vi "WaveFormnew.vi"(11 "2D Double Array 3":i32[][](array[numeric])) -> (1 "2D Double Array":i32[](array[numeric]), 2 "Waveform Chart 3":waveform(i32)[](graph) caption="Waveform Chart 2", 3 "2D Double Array 2":i32[][](array[numeric]), 4 "Waveform Chart":waveform(i32)(graph), 5 "XY Graph":cluster{i32[], u64[]}(graph))   [LabVIEW 2023]
uses:
  <vilib>/numeric/Random Number (Range) U64.vi
  <vilib>/numeric/sub_Random U32.vi
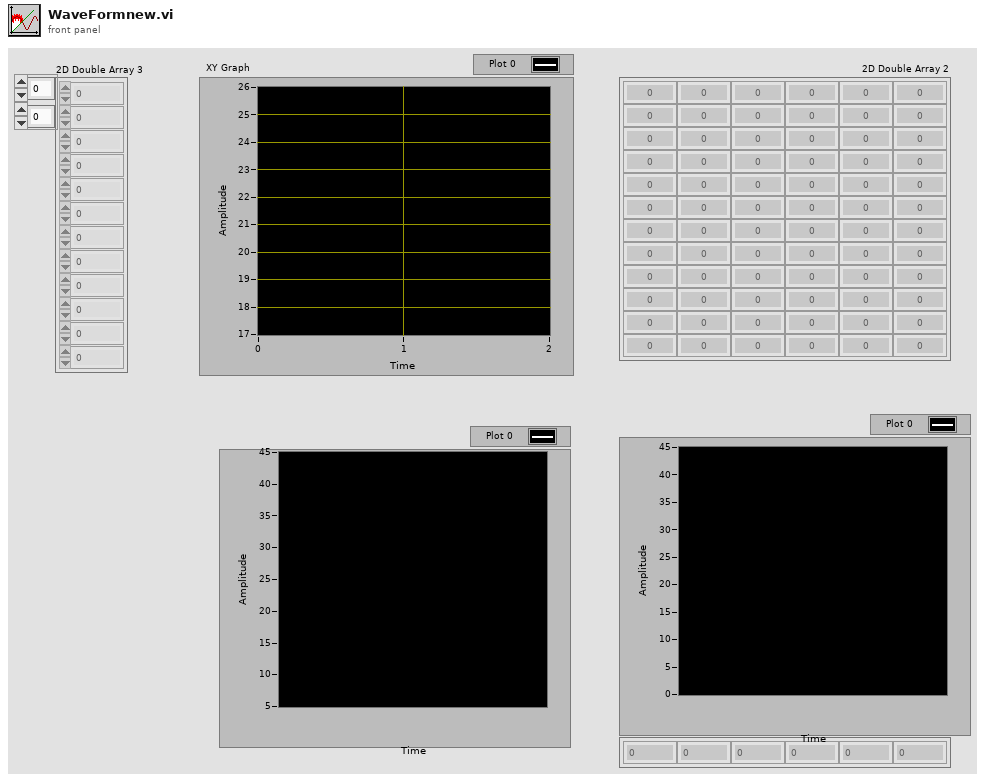
[diagram p1: front panel]
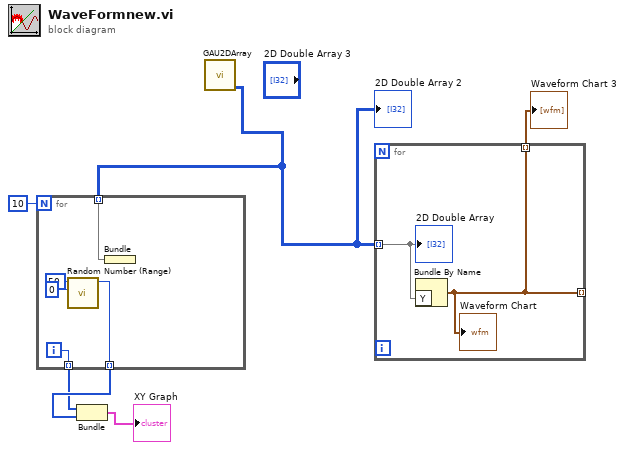
[diagram p0: block diagram]
diagram:
  n1 = call "GAU2DArray.vi"() -> ("2D Double Array"=w1:i32[][])  [unwired: 10 in, 1 out]
  "2D Double Array 2" <- w1
  n2 = for {
    N: 10 -> [_]
    tunnel: w1 -> [w11] mode=indexing
    tunnel: [w10] -> w3 mode=indexing
    tunnel: [w7] -> w4 mode=indexing
    i -> [w10]
    n3 = call-poly <vilib>:"Random Number (Range).vi"("lower bound (0)"=u64 0, "upper bound (100)"=u64 50) -> ("number"=w7:u64)  [unwired: 9 in]
    n4 = Bundle("2D Double Array"=w11) -> ()  [unwired: 1 in, 1 out]
  }
  n5 = Bundle(w3, w4) -> (→"XY Graph":cluster{i32[], u64[]})  [unwired: 1 in]
  n6 = for {
    tunnel: w1 -> [w13] mode=indexing
    tunnel: [w12] -> _ mode=indexing
    tunnel: [w12] -> w2 mode=indexing
    n7 = Bundle By Name("Y"=w13) -> (w12:waveform(i32))  [unwired: 1 in]
    "Waveform Chart" <- w12
    "2D Double Array" <- w13
  }
  "Waveform Chart 3" <- w2
